vi "ACT_7_Task1_vikas.potluri.vi"() -> ()   [LabVIEW 2016]
panel:
  out "Numeric 3":dbl
  in  "Numeric 2":dbl
  in  "Numeric":dbl
  in  "Radio Buttons":T1(radio)
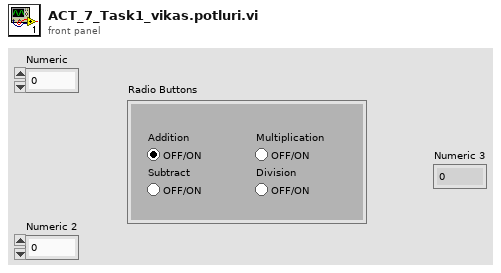
[diagram p1: front panel]
types:
  T1 = enum32{"Addition", "Subtract", "Division", "Multiplication"}
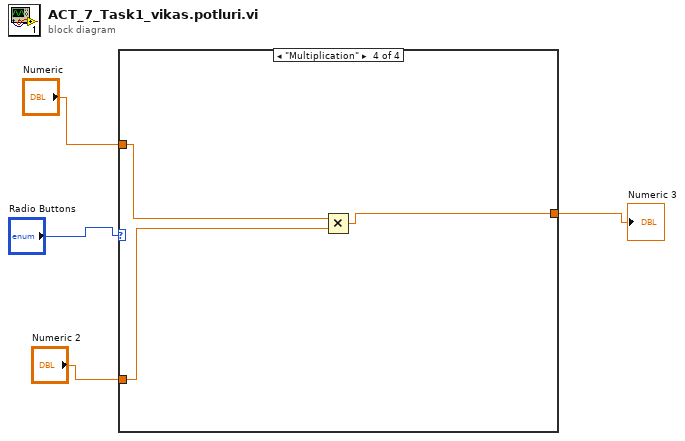
[diagram p0: block diagram]
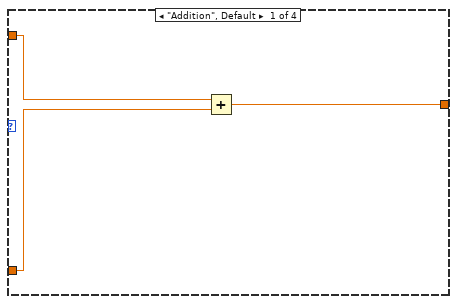
[diagram p2: hidden frame]
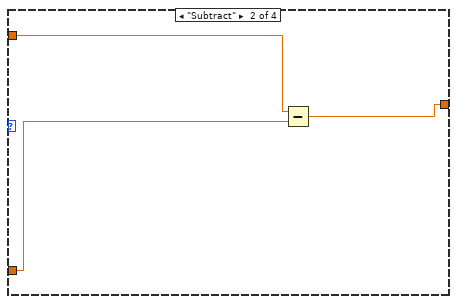
[diagram p3: hidden frame]
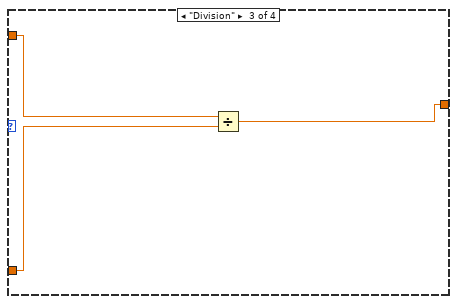
[diagram p4: hidden frame]
diagram:
  n1 = case shown="\"Multiplication\"" "Radio Buttons" {
    tunnel: "Numeric 2" -> [w6 w8 w12 w15]
    tunnel: "Numeric" -> [w7 w9 w13 w16]
    tunnel: [w5 w10 w11 w14] -> w1
    frame "Addition", Default {
      n2 = Add(x=w7, y=w6) -> (x+y=w5:dbl)
    }
    frame "Subtract" {
      n3 = Subtract(x=w9, y=w8) -> (x-y=w10:dbl)
    }
    frame "Division" {
      n4 = Divide(x=w13, y=w12) -> (x/y=w11:dbl)
    }
    frame "Multiplication" {
      n5 = Multiply(x=w16, y=w15) -> (x*y=w14:dbl)
    }
  }
  "Numeric 3" <- w1
